vi "PH_BeamlineController.PC calc Synchrolock.vi"(0 "i ref in":refnum<vi>, 5 "error in":errorcluster) -> (14 "i ref out":refnum<vi>, 19 "error out":errorcluster)   [LabVIEW 2014, in "PH_BeamlineController.lvlib"]
doc: "This VI indicates the status of the fs Synchrolock if it is of interest."
uses:
  PH_BeamlineController.lvlib
  PH_Beamline_Chief/PH_Beamline_Chief.Section.ctl
  PH_Common/PH_Common.lvlib
  PH_Beamline_Chief/PH_Beamline_Chief.lvlib
  PH_BeamlineInformation/PH_BeamlineInformation.lvlib
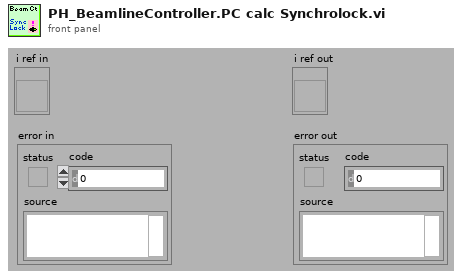
[diagram p1: front panel]
types:
  T1 = typedef "PH_Beamline_Chief.lvlib/PH_Beamline_Chief.Section.ctl" = enum16{"None", "YLF", "fs", "fs-YLF", "ns", "PA-Input", "PA-Undelay", "PA-Delay", "PA-before-Bypass", "PA", "PA-Bypass", "PA-Exit", "PA-LL", "LL", "PA-MA", "MA-Exit", "MA-Z6", "Z6", "MA-LB", "LB-TB2", "LB-TB3"}
  T2 = typedef "PH_StatusHandler.lvlib/PH_StatusHandler.Status.ctl" = i16
  T3 = typedef "PH_BeamlineController.lvlib/PH_BeamlineController.i attribute.ctl" = cluster{"Vacuum Exp LB":cluster{"Channel":string, "Limit [mbar]":dbl, "Pressure [mbar]":dbl, "GUI Ref":refnum<vi>}, "Sources":T4[], "PA DP Targets":T6[], "Path":cluster{"Source":T5, "PA DP Target":T7, "Target":T8}, "Targets":cluster{"Name":T8, "GUI Ref":refnum<vi>, "Current State":bool, "Wanted State":bool, "Enabled":bool}[], "Status Tags":cluster{"Name":string, "Status":T2}[], "special GUI Refs":T9}
  T4 = typedef "PH_BeamlineController.lvlib/PH_BeamlineController.Source Attributes.ctl" = cluster{"Name":T5, "GUI Ref":refnum<vi>, "Current State":bool, "Wanted State":bool}
  T5 = typedef "PH_BeamlineController.lvlib/PH_BeamlineController.Sources.ctl" = enum16{"None", "YLF", "fs-Frontend", "ns-Frontend", "YLF and ns-Frontend", "fs- and ns-Frontend"}
  T6 = typedef "PH_BeamlineController.lvlib/PH_BeamlineController.PA DP Target Attributes.ctl" = cluster{"Name":T7, "GUI Ref":refnum<vi>, "Current State":bool, "Wanted State":bool, "Enabled":bool}
  T7 = typedef "PH_BeamlineController.lvlib/PH_BeamlineController.PA DP Targets.ctl" = enum16{"None", "Dump PA Delayed Beam", "Dump PA Undelayed Beam", "Dumps PA Delayed and Undelayed Beam"}
  T8 = typedef "PH_BeamlineController.lvlib/PH_BeamlineController.Targets.ctl" = enum16{"None", "PreAmp", "Dump Exp Laserlab", "Exp Laserlab", "Calorimeter", "Dump Exp Laserbay", "Exp Laserbay", "Dump Exp Z6", "Exp Z6"}
  T9 = typedef "PH_BeamlineController.lvlib/PH_BeamlineController.special GUI Refs.ctl" = cluster{"PA-Backreflection-Meas":refnum<vi>, "fs_Synchrolock_Watch":refnum<vi>}
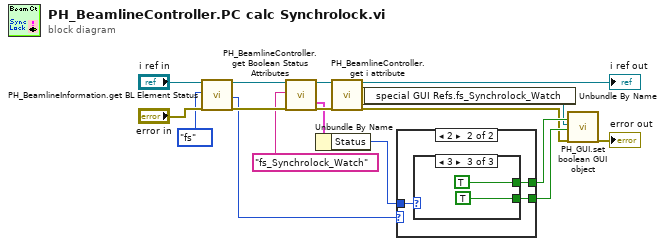
[diagram p0: block diagram]
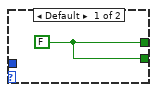
[diagram p2: hidden frame]
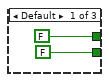
[diagram p3: hidden frame]
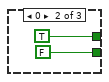
[diagram p4: hidden frame]
diagram:
  n1 = call "PH_BeamlineInformation.get BL Element Status.vi"("VI in"="i ref in", "Beamline Element"=PH_Beamline_Chief.Section."fs" ("Beamline Section"), "error in (no error)"="error in") -> ("VI out"=w11:refnum<vi>, "Status"=w9:i32, "error out"=w13:errorcluster)  [unwired: 14 in]
  n2 = call "PH_BeamlineController.get Boolean Status Attributes.vi"("VI in"=w11, "Name"="fs_Synchrolock_Watch" ("Synchrolock.Instance"), "error in (no error)"=w13) -> ("VI out"=w4:refnum<vi>, "Tag"=w8:cluster{"Name":string, "Status":T2}, "error out"=w15:errorcluster)  [unwired: 11 in, 3 out]
  n3 = Unbundle By Name(w8) -> ("Status"=w7:T2)
  n4 = call "PH_BeamlineController.get i attribute.vi"("i ref in"=w4, "error in (no error)"=w15) -> ("i ref out"=→"i ref out":refnum<vi>, "i attribute"=w2:T3, "error out"=w5:errorcluster)  [unwired: 15 in]
  n5 = Unbundle By Name(w2) -> ("special GUI Refs.fs_Synchrolock_Watch"=w1:refnum<vi>)
  n6 = case shown="2" w9 {
    tunnel: w7 -> [_ w22]
    tunnel: [w19 w21] -> w17
    tunnel: [w19 w20] -> w16
    frame Default {
      w19 = FALSE
    }
    frame 2 {
      n7 = case shown="3" w22 {
        tunnel: [FALSE TRUE TRUE] -> w21
        tunnel: [FALSE FALSE TRUE] -> w20
        frame Default {
        }
        frame 0 {
        }
        frame 3 {
        }
      }
    }
  }
  n8 = call "PH_GUI.set boolean GUI object.vi"("Visible (true)"=w17, "Boolean Knob GUI Ref"=w1, "Value"=w16, "error in (no error)"=w5) -> ("error out"=→"error out":errorcluster)  [unwired: 15 in]
